vi "channelScan.vi"() -> ()   [LabVIEW 2016]
uses:
  <vilib>/Analysis/Matrix/Datatypes/RealMatrix.ctl
  <vilib>/Utility/file.llb/Write Delimited Spreadsheet (DBL).vi
  <vilib>/Analysis/Matrix/NI_Matrix.lvlib
panel:
  in  "测量最大电压":dbl=16.0 min=1.0 max=1000.0 step=1.0
  in  "通道数":i16=64 min=1 max=1000 step=1
  in  "HIFU":refnum<visa-resource-name>
  in  "Real Matrix":T1
  out "voltage":dbl
  out "channel":dbl
  in  "Start":bool
  in  "osc in":refnum<visa-resource-name>
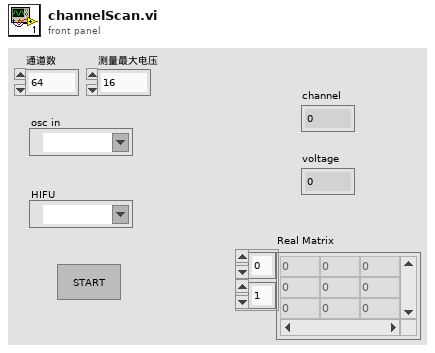
[diagram p1: front panel]
types:
  T1 = typedef "NI_Matrix.lvlib/RealMatrix.ctl" = dbl[][]
  T2 = enum16{"open", "replace", "create", "open or create", "replace or create", "replace or create with confirmation"}
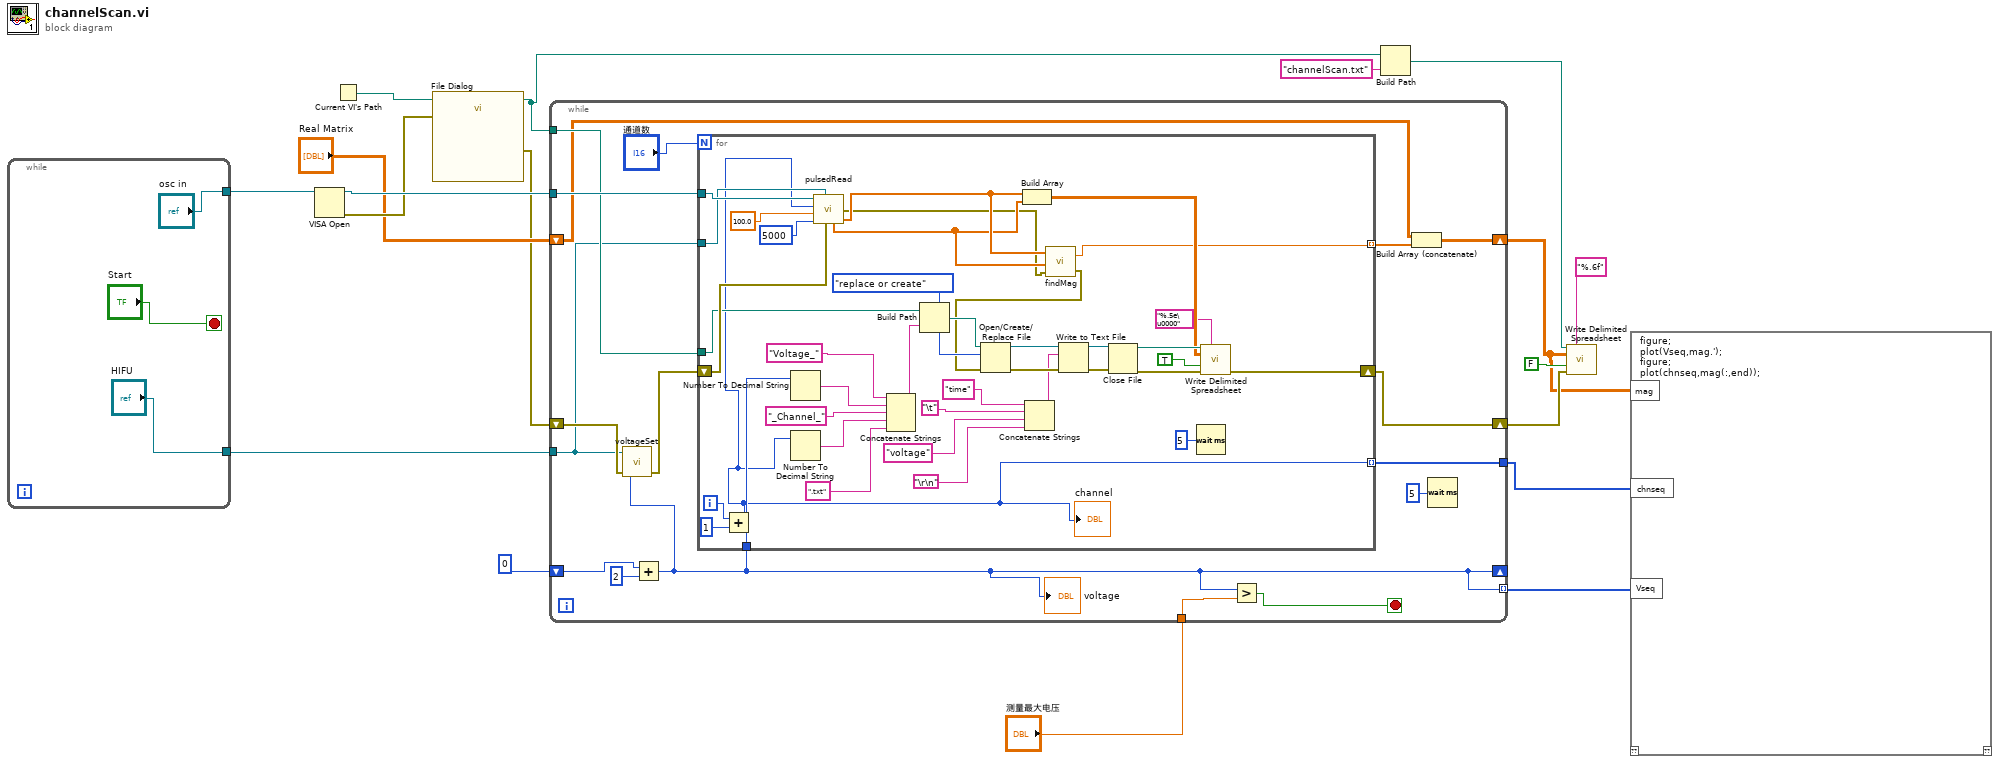
[diagram p0: block diagram]
diagram:
  n1 = while {
    tunnel: ["osc in"] -> w18
    tunnel: ["HIFU"] -> w5
    stop <- "Start" stop-if-true
  }
  n2 = VISA Open(VISA resource name=w18) -> (VISA resource name=w16:refnum<visa-resource-name>, error out=w14:errorcluster)  [unwired: 4 in]
  n3 = Current VI's Path() -> (path=w15:path)
  n4 = call "File Dialog"("start path"=w15, "error in"=w14) -> ("selected path"=w9:path, "error out"=w6:errorcluster)  [unwired: 10 in, 2 out]
  n5 = while {
    shift-right: [w23] -> _
    shift-left: 0 -> [w38]
    tunnel: w16 -> [w34]
    tunnel: w9 -> [w33]
    shift-right: [w30] -> w1
    shift-left: "Real Matrix" -> [w29]
    shift-right: [w28] -> w11
    shift-left: w6 -> [w36]
    tunnel: w5 -> [w26]
    tunnel: "测量最大电压" -> [w25]
    tunnel: [w23] -> w3 mode=indexing
    tunnel: [w22] -> w2
    stop <- w32 stop-if-true
    n6 = Add(x=w38, y=2) -> (x+y=w23:i32)
    "voltage" <- w23
    n7 = call "voltageSet.vi"("error in (no error)"=w36, "Voltage"=w23, "HIFU UART in"=w26) -> ("error out"=w35:errorcluster)  [unwired: 2 out]
    n8 = for {
      N: "通道数" -> [_]
      tunnel: w34 -> [w77]
      tunnel: w33 -> [w67]
      tunnel: w23 -> [w73]
      shift-right: [w50] -> w28
      shift-left: w35 -> [w74]
      tunnel: [w47] -> w31 mode=indexing
      tunnel: w26 -> [w42]
      tunnel: [w39] -> w22 mode=indexing
      i -> [w41]
      n9 = Add(x=w41, y=1) -> (x+y=w39:i32)
      "channel" <- w39
      n10 = Number To Decimal String(number=w73) -> (decimal integer string=w71:string)  [unwired: 1 in]
      n11 = Number To Decimal String(number=w39) -> (decimal integer string=w69:string)  [unwired: 1 in]
      n12 = call "pulsedRead.vi"("error in (no error)"=w74, "points"=u64 5000, "cycles"=100.0, "HIFU UART in"=w42, "channel"=w39, "osc in"=w77) -> ("time"=w46:dbl[], "voltage"=w45:dbl[], "error out"=w44:errorcluster)  [unwired: 2 out]
      n13 = Concatenate Strings("Voltage_", w71, "_Channel_", w69, ".txt") -> (w66:string)
      n14 = Build Path(base path=w67, name or relative path=w66) -> (appended path=w65:path)
      n15 = Build Array(w46, w45) -> (w53:T1)
      n16 = Concatenate Strings("time", "\t", "voltage" ("string"), "\r\n") -> (w58:string)
      n17 = call "findMag.vi"("error in (no error)"=w44, "voltages"=w45, "times"=w46) -> ("error out"=w43:errorcluster, "magfound"=w47:dbl)
      n18 = Open/Create/Replace File(file path (use dialog)=w65, error in=w43, operation (0:open)=T2."replace or create") -> (refnum out=w57:refnum<file>, error out=w63:errorcluster)  [unwired: 3 in, 1 out]
      n19 = Write to Text File(file (use dialog)=w57, text=w58, error in=w63) -> (refnum out=w55:refnum<file>, error out=w56:errorcluster)  [unwired: 1 in, 1 out]
      n20 = Close File(refnum=w55, error in=w56) -> (path=w54:path, error out=w51:errorcluster)
      n21 = Wait (ms)(milliseconds to wait=u32 5) -> ()  [unwired: 1 out]
      n22 = call-poly <vilib>:"Write Delimited Spreadsheet.vi"("file path (dialog if empty)"=w54, "format (%.3f)"="%.5e\u0000", "2D data"=w53, "append to file? (new file:F)"=TRUE, "error in (no error)"=w51) -> ("error out"=w50:errorcluster)  [unwired: 9 in, 1 out]
    }
    n23 = Greater?(x=w23, y=w25) -> (0:w32:bool)
    n24 = Build Array (concatenate)(w29, w31) -> (w30:T1)
    n25 = Wait (ms)(milliseconds to wait=u32 5) -> ()  [unwired: 1 out]
  }
  n26 = Build Path(base path=w9, name or relative path="channelScan.txt") -> (appended path=w8:path)
  n27 = call-poly <vilib>:"Write Delimited Spreadsheet.vi"("file path (dialog if empty)"=w8, "format (%.3f)"="%.6f", "2D data"=w1, "append to file? (new file:F)"=FALSE, "error in (no error)"=w11) -> ()  [unwired: 9 in, 2 out]
  n28 = script code="figure;\nplot(Vseq,mag.');\nfigure;\nplot(chnseq,mag(:,end));"("Vseq"=w3, "chnseq"=w2, "mag"=w1) -> ()  [unwired: 1 in, 1 out]
